vi "Update Device Status.vi"(8 "error in":errorcluster, 11 "Manual Control in":refnum<class "Manual Control.lvclass">) -> (0 "error out":errorcluster, 3 "Manual Control out":refnum<class "Manual Control.lvclass">)   [LabVIEW 2018, in "Manual Control Actor.lvlib" / "Manual Control.lvclass"]
uses:
  Manual Control.lvclass
  C:/Users/Administrator/Desktop/2018LabVIEW EMS/EMS Generic Actor/EMS Generic/EMS Generic.lvclass
  C:/Program Files (x86)/National Instruments/LabVIEW 2018/vi.lib/ActorFramework/Actor/Actor.lvclass
  Manual Control.lvclass/Manual Control.ctl
  <vilib>/ActorFramework/Actor/Actor.lvclass/Actor.ctl
  EMS Generic Actor/EMS Generic/EMS Generic.lvclass/EMS Generic.ctl
  EMS Generic Actor/EMS Generic Messages/Return IED_Status Msg/Return IED_Status Msg.lvclass/Return IED_Status Msg.ctl
  <vilib>/ActorFramework/Message Enqueuer/Message Enqueuer.lvclass/Message Enqueuer.ctl
  <vilib>/ActorFramework/Message Enqueuer/Enqueue.vi
  EMS Generic Actor/EMS Generic Messages/Return IED_Status Msg/Return IED_Status Msg.lvclass
  C:/Program Files (x86)/National Instruments/LabVIEW 2018/vi.lib/ActorFramework/Message/Message.lvclass
  <vilib>/ActorFramework/Message Priority Queue/Priority Enqueue.vi
  <vilib>/ActorFramework/Actor/Actor.lvclass
  EMS Generic Actor/EMS Generic/EMS Generic.lvclass
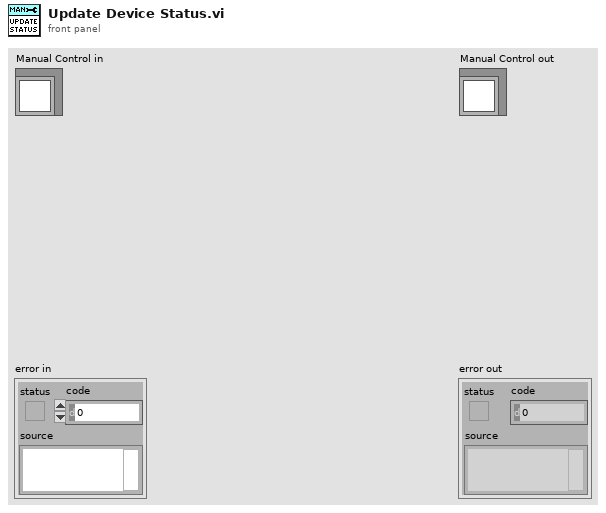
[diagram p1: front panel]
types:
  T1 = typedef "CSEISMIC DDS.lvlib/CSEISMIC DDS.lvclass/DeviceID.ctl" = string
  T2 = typedef "CSEISMIC DDS.lvlib/CSEISMIC DDS.lvclass/IED_Status.ctl" = cluster{"DeviceID":T1, "Timestamp":T3, "MicrogridID":u8, "Active":bool, "Inactive":bool, "Error":i32, "Fault":bool, "ErrorString":string}
  T3 = typedef "CSEISMIC DDS.lvlib/CSEISMIC DDS.lvclass/Timestamp.ctl" = cluster{"Seconds":u64, "Remainder":u64}
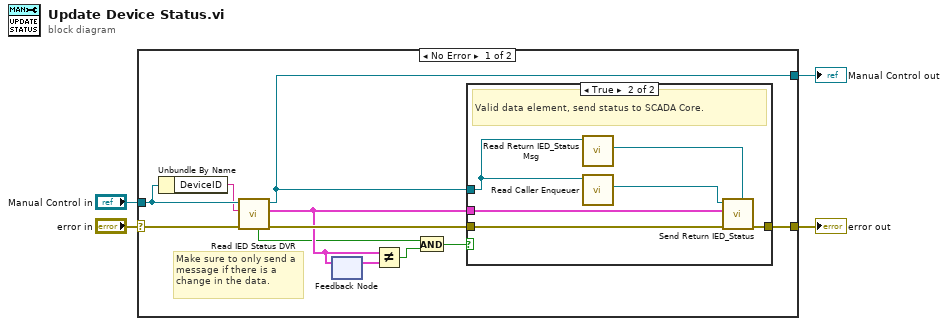
[diagram p0: block diagram]
diagram:
  n1 = case shown="No Error" "error in" {
    selector: "error in" -> [w13 w24]
    tunnel: [w10 w24] -> w3
    tunnel: [w12 w23] -> w1
    tunnel: "Manual Control in" -> [w15 w23]
    frame No Error {
      # "Make sure to only send a message if there is a change in the data."
      n2 = Unbundle By Name(w15) -> ("DeviceID"=w14:T1)
      n3 = call "Read IED Status DVR.vi"("error in"=w13, "DeviceID"=w14, "EMS Generic in"=w15) -> ("error out"=w11:errorcluster, "IED_Status"=w7:T2, "EMS Generic out"=w12:refnum<class "Manual Control.lvclass">, "valid?"=w6:bool)  [unwired: 5 in]
      n4 = feedback #1() -> (w9:T2)  [unwired: 1 in]
      n5 = feedback-in #1(w7) -> ()
      n6 = Not Equal?(x=w7, y=w9) -> (x != y?=w8:bool)
      n7 = And(x=w6, y=w8) -> (x .and. y?=w5:bool)
      n8 = case shown="True" w5 {
        tunnel: w12 -> [_ w22]
        tunnel: w7 -> [_ w19]
        tunnel: w11 -> [w16 w21]
        tunnel: [w16 w20] -> w10
        frame False {
          # "#TODO Should update status on Master Controller Core"
          # "No IED_Status data available for specified device"
        }
        frame True {
          # "Valid data element, send status to SCADA Core."
          n9 = call "Read Return IED_Status Msg.vi"("EMS Generic in"=w22) -> ("Return IED_Status Msg"=w17:refnum<class "Return IED_Status Msg.lvclass">)  [unwired: 9 in, 1 out]
          n10 = call <vilib>:"Read Caller Enqueuer.vi"("Actor"=w22) -> ("Caller Enqueuer"=w18:refnum<class "Message Enqueuer.lvclass">)  [unwired: 10 in]
          n11 = call "Send Return IED_Status.vi"("Message Type"=w17, "error in (no error)"=w21, "IED_Status"=w19, "Message Enqueuer"=w18) -> ("error out"=w20:errorcluster)  [unwired: 6 in, 1 out]
        }
      }
    }
    frame Error {
    }
  }
  "error out" <- w3
  "Manual Control out" <- w1
